vi "Rename and Refactor Dependency for Object.vi"(8 "error in (no error)":errorcluster, 10 "rename data":T2, 11 "object references":refnum<vi>[](array[refnum])) -> (0 "error out":errorcluster, 2 "refactor results":T1[](array[typedef]))   [LabVIEW 2020, in "MeasurementService Editor.lvlib"]
uses:
  MeasurementService Editor.lvlib
  Rename Refactor Data.ctl
  Rename Refactor Mapping Info.ctl
  Refactor Object Result.ctl
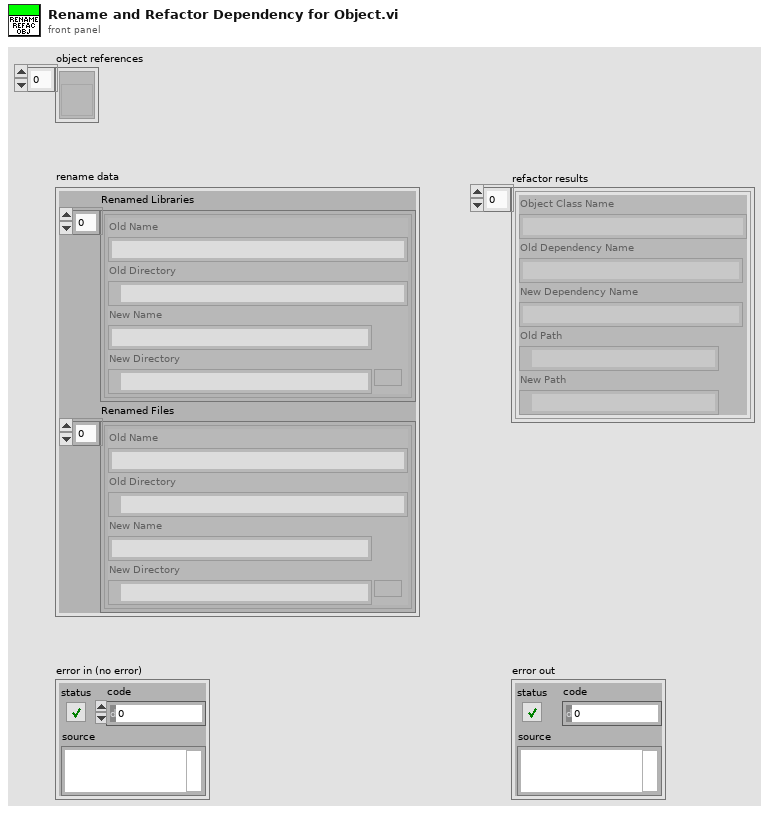
[diagram p1: front panel]
types:
  T1 = typedef "MeasurementService Editor.lvlib/Refactor Object Result.ctl" = cluster{"Object Class Name":string, "Old Dependency Name":string, "New Dependency Name":string, "Old Path":path, "New Path":path}
  T2 = typedef "MeasurementService Editor.lvlib/Rename Refactor Data.ctl" = cluster{"Renamed Libraries":T3[], "Renamed Files":T3[]}
  T3 = typedef "MeasurementService Editor.lvlib/Rename Refactor Mapping Info.ctl" = cluster{"Old Name":string, "Old Directory":path, "New Name":string, "New Directory":path}
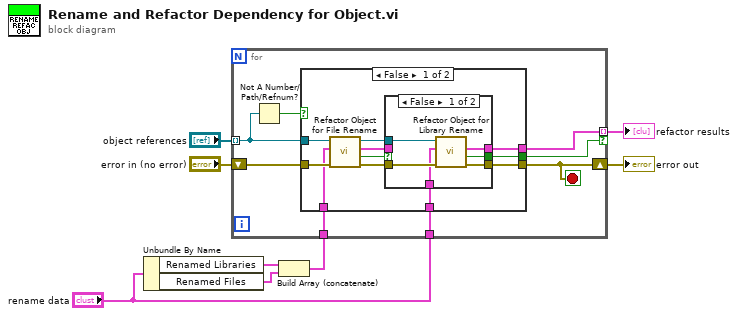
[diagram p0: block diagram]
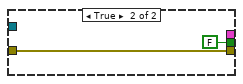
[diagram p3: hidden frame]
diagram:
  n1 = Unbundle By Name("rename data") -> ("Renamed Libraries"=w3:T3[], "Renamed Files"=w2:T3[])
  n2 = Build Array (concatenate)(w3, w2) -> (w1:T3[])
  n3 = for {
    tunnel: "object references" -> [w11] mode=indexing
    shift-right: [w15] -> w8
    shift-left: "error in (no error)" -> [w16]
    tunnel: [w14] -> w5 mode=indexing if=w13
    tunnel: "rename data" -> [w12]
    tunnel: w1 -> [w9]
    stop <- w15 stop-if-true
    n4 = Not A Number/Path/Refnum?(number/path/refnum=w11) -> (NaN/Path/Refnum?=w10:bool)
    n5 = case shown="False" w10 {
      tunnel: w16 -> [w27 w38]
      tunnel: [w23 w38] -> w15
      tunnel: [w21 _] -> w14
      tunnel: [w20 FALSE ("refactored dependency")] -> w13
      tunnel: w12 -> [w19 _]
      tunnel: w11 -> [w18 _]
      tunnel: w9 -> [w17 _]
      frame False {
        n6 = call "Refactor Object for File Rename.vi"("error in (no error)"=w27, "renamed files"=w17, "object reference in"=w18) -> ("error out"=w24:errorcluster, "refactored dependency"=w26:bool, "refactor result"=w22:T1, "object reference out"=w25:refnum<vi>)  [unwired: 5 in]
        n7 = case shown="False" w26 {
          selector: w26 -> [_ w34]
          tunnel: w25 -> [w33 _]
          tunnel: w24 -> [w32 w35]
          tunnel: [w31 w35] -> w23
          tunnel: w22 -> [_ w36]
          tunnel: [w30 w36] -> w21
          tunnel: [w29 w34] -> w20
          tunnel: w19 -> [w28 _]
          frame False {
            n8 = call "Refactor Object for Library Rename.vi"("error in (no error)"=w32, "rename data"=w28, "object reference in"=w33) -> ("error out"=w31:errorcluster, "refactored dependency"=w29:bool, "refactor result"=w30:T1)  [unwired: 5 in, 1 out]
          }
          frame True {
          }
        }
      }
      frame True {
      }
    }
  }
  "error out" <- w8
  "refactor results" <- w5
